vi "Launch_HMI.vi"(8 "error in (no error)":errorcluster caption="entrée d'erreur (pas d'erreur)", 11 "Class Popup (Default) en entrée":refnum<class "Class Popup Operator_Input_PCRE.lvclass">) -> (0 "error out":errorcluster caption="sortie d'erreur", 3 "Class Popup (Default) en sortie":refnum<class "Class Popup Operator_Input_PCRE.lvclass">)   [LabVIEW 2020, in "Library Instrument & Equipement.lvlib" / "Library Popup.lvlib" / "Class Popup Operator_Input_PCRE.lvclass"]
uses:
  Class Popup Operator_Input_PCRE.lvclass
  Class Popup (Main)/Class Popup (Main).lvclass
  Class Popup Operator_Input_PCRE.lvclass/Class Popup Operator_Input_PCRE.ctl
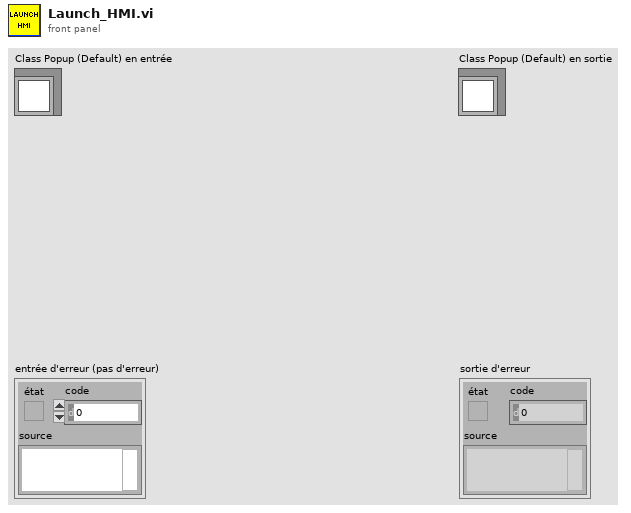
[diagram p1: front panel]
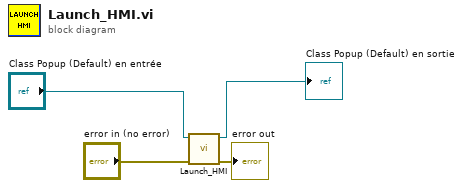
[diagram p0: block diagram]
diagram:
  n1 = call-parent "Launch_HMI.vi"("error in (no error)"="error in (no error)", "Class Popup (Default) en entrée"="Class Popup (Default) en entrée") -> ("error out"=→"error out":errorcluster, "Class Popup (Default) en sortie"=→"Class Popup (Default) en sortie":refnum<class "Class Popup Operator_Input_PCRE.lvclass">)  [unwired: 8 in]
